vi "BasicExampleMux.vi"() -> ()   [LabVIEW 2025]
uses:
  PalmSens/PalmSens.lvclass
  C:/Users/stef/code/palmsenssdk/labview/PalmSens/Libraries/PalmSens.Core.Simplified.LabVIEW.dll
  PalmSens/Libraries/PalmSens.Core.Simplified.LabVIEW.dll
  PalmSens/MeasurementResults.ctl
  PalmSens/LiveCurveResult.ctl
panel:
  out "BitArray out":bool[](array[boolean])
  in  "Mux channels":bool[](array[boolean])
  out "Results":T1
  out "LSV Method Indicator":refnum<k24>
  out "Array":string[](array[string])
  out "Is Measuring":bool
  in  "PalmSens.lvclass":refnum<class "PalmSens.lvclass">
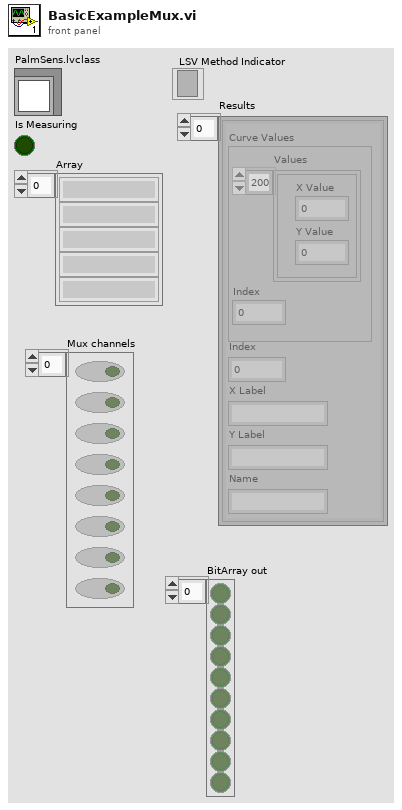
[diagram p1: front panel]
types:
  T1 = typedef "MeasurementResults.ctl" = T2[]
  T2 = typedef "LiveCurveResult.ctl" = cluster{"X Label":string, "Y Label":string, "Name":string, "Index":i16, "Curve Values":cluster{"Values":cluster{"X Value":dbl, "Y Value":dbl}[], "Index":i16}}
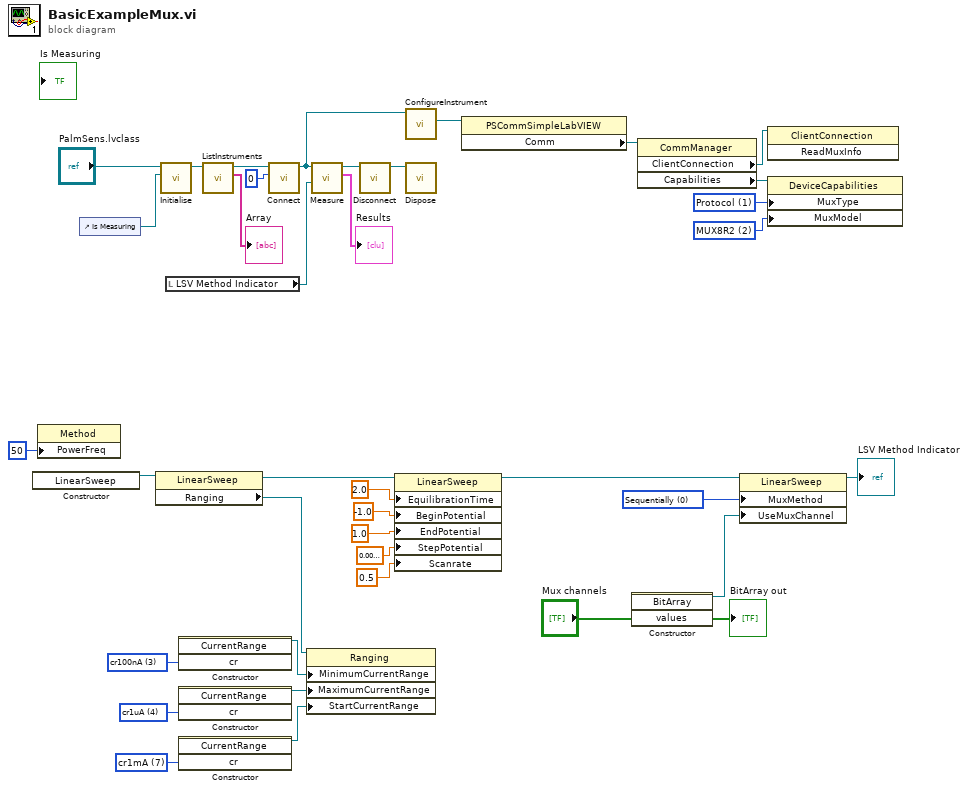
[diagram p0: block diagram]
diagram:
  w12 = 2 items=["MUX8", "MUX16", "MUX8R2", "PicoMUX16", "PicoMUX256"] ("MuxModel")
  w15 = 0 items=["Sequentially"=0, "Alternatingly"=1, "None"=-1] ("MuxMethod")
  w18 = 1 items=["AuxAddress", "Protocol"] ("MuxType")
  w27 = 4 items=["cr100pA"=0, "cr1nA"=1, "cr10nA"=2, "cr100nA"=3, "cr1uA"=4, "cr10uA"=5, "cr100uA"=6, "cr1mA"=7, "cr10mA"=8, "cr100mA"=9, "cr2uA"=10, "cr4uA"=11, "cr8uA"=12, "cr16uA"=13, "cr32uA"=14, "cr125uA"=17, "cr250uA"=18, "cr500uA"=19, "cr5mA"=20, "cr6uA"=21, "cr13uA"=22, "cr25uA"=23, "cr50uA"=24, "cr200uA"=25, "cr63uA"=26] ("cr")
  w28 = 7 items=["cr100pA"=0, "cr1nA"=1, "cr10nA"=2, "cr100nA"=3, "cr1uA"=4, "cr10uA"=5, "cr100uA"=6, "cr1mA"=7, "cr10mA"=8, "cr100mA"=9, "cr2uA"=10, "cr4uA"=11, "cr8uA"=12, "cr16uA"=13, "cr32uA"=14, "cr125uA"=17, "cr250uA"=18, "cr500uA"=19, "cr5mA"=20, "cr6uA"=21, "cr13uA"=22, "cr25uA"=23, "cr50uA"=24, "cr200uA"=25, "cr63uA"=26] ("cr")
  w30 = 3 items=["cr100pA"=0, "cr1nA"=1, "cr10nA"=2, "cr100nA"=3, "cr1uA"=4, "cr10uA"=5, "cr100uA"=6, "cr1mA"=7, "cr10mA"=8, "cr100mA"=9, "cr2uA"=10, "cr4uA"=11, "cr8uA"=12, "cr16uA"=13, "cr32uA"=14, "cr125uA"=17, "cr250uA"=18, "cr500uA"=19, "cr5mA"=20, "cr6uA"=21, "cr13uA"=22, "cr25uA"=23, "cr50uA"=24, "cr200uA"=25, "cr63uA"=26] ("cr")
  n1 = constructor class="LinearSweep"() -> (reference out=w32:refnum<k24>)  [unwired: 3 in, 2 out]
  n2 = property class="Method"("PowerFreq"=50) -> ()  [unwired: 2 in, 2 out]
  n3 = control-ref of="Is Measuring"() -> (w37:refnum<vi>)
  n4 = property class="LinearSweep"(reference=w32) -> (reference out=w26:refnum<k24>, "Ranging"=w31:refnum<k24>)  [unwired: 1 in, 1 out]
  n5 = call-dynamic "Initialise.vi"("Is Measuring Refnum"=w37, "PalmSens in"="PalmSens.lvclass") -> ("PalmSens out"=w36:refnum<class "PalmSens.lvclass">)  [unwired: 8 in, 1 out]
  n6 = local read "LSV Method Indicator"() -> (w20:refnum<k24>)
  n7 = constructor class="CurrentRange"("cr"=w30) -> (reference out=w29:refnum<k24>)  [unwired: 3 in, 3 out]
  n8 = constructor class="CurrentRange"("cr"=w27) -> (reference out=w9:refnum<k24>)  [unwired: 3 in, 3 out]
  n9 = constructor class="CurrentRange"("cr"=w28) -> (reference out=w8:refnum<k24>)  [unwired: 3 in, 3 out]
  n10 = call-dynamic "ListInstruments.vi"("PalmSens in"=w36) -> ("Array"=→"Array":string[], "PalmSens out"=w34:refnum<class "PalmSens.lvclass">)  [unwired: 8 in, 1 out]
  n11 = call-dynamic "Connect.vi"("Instrument Index"=0, "PalmSens in"=w34) -> ("PalmSens out"=w17:refnum<class "PalmSens.lvclass">)  [unwired: 8 in, 1 out]
  n12 = property class="Ranging"(reference=w31, "MinimumCurrentRange"=w29, "MaximumCurrentRange"=w9, "StartCurrentRange"=w8) -> ()  [unwired: 1 in, 2 out]
  n13 = call-dynamic "Measure.vi"("Method .NET Refnum"=w20, "PalmSens in"=w17) -> ("Curves"=→"Results":T1, "PalmSens out"=w21:refnum<class "PalmSens.lvclass">)  [unwired: 2 in, 2 out]
  n14 = call-dynamic "Disconnect.vi"("PalmSens in"=w21) -> ("PalmSens out"=w23:refnum<class "PalmSens.lvclass">)  [unwired: 9 in, 1 out]
  n15 = property class="LinearSweep"(reference=w26, "EquilibrationTime"=sgl 2.0, "BeginPotential"=sgl -1.0, "EndPotential"=sgl 1.0, "StepPotential"=sgl 0.01, "Scanrate"=sgl 0.5) -> (reference out=w7:refnum<k24>)  [unwired: 1 in, 1 out]
  n16 = call-dynamic "ConfigureInstrument.vi"("PalmSens in"=w17) -> ("PSLabView Instance"=w16:refnum<k24>)  [unwired: 8 in, 2 out]
  n17 = call-dynamic "Dispose.vi"("PalmSens in"=w23) -> ()  [unwired: 9 in, 2 out]
  n18 = property class="PSCommSimpleLabVIEW"(reference=w16) -> ("Comm"=w19:refnum<k24>)  [unwired: 1 in, 2 out]
  n19 = constructor class="BitArray"("values"="Mux channels") -> (reference out=w11:refnum<k24>, "values"=→"BitArray out":bool[])  [unwired: 3 in, 2 out]
  n20 = property class="CommManager"(reference=w19) -> ("ClientConnection"=w1:refnum<k24>, "Capabilities"=w2:refnum<k24>)  [unwired: 1 in, 2 out]
  n21 = property class="LinearSweep"(reference=w7, "MuxMethod"=w15, "UseMuxChannel"=w11) -> (reference out=→"LSV Method Indicator":refnum<k24>)  [unwired: 1 in, 1 out]
  n22 = invoke class="ClientConnection" method="ReadMuxInfo"(reference=w1) -> ()  [unwired: 2 in, 3 out]
  n23 = property class="DeviceCapabilities"(reference=w2, "MuxType"=w18, "MuxModel"=w12) -> ()  [unwired: 1 in, 2 out]
